vi "RT Main R2.vi"() -> ()   [LabVIEW 2018]
uses:
  Type Defs/Control Mode Type Def.ctl
  Type Defs/Sine Wave Inputs.ctl
  Type Defs/Measurement States.ctl
  <vilib>/Platform/TimedLoop/XDataNode/timing_clust.ctl
  <vilib>/Platform/TimedLoop/XDataNode/nitl_modes.ctl
  <vilib>/Platform/TimedLoop/XDataNode/wakeup.ctl
  Type Defs/PID Inputs.ctl
  <vilib>/FPGAPlugInAG/myRIO-1900/niLvFpga_Open_myRIO-1900.vi
  <vilib>/rvi/interface/common/dynamic/niFpgaDynamicAddResources.vi
  <vilib>/Utility/error.llb/Error Cluster From Error Code.vi
  <vilib>/rvi/errors/niLvFpgaAdjustHostInterfaceError.vi
  <vilib>/addons/control/pid/pid.llb/PID (DBL).vi
  <vilib>/FPGAPlugInAG/Dynamic/niLvFpga_Close_Dynamic.vi
  <vilib>/platform/TimedLoop/XDataNode/XDataNode.xnode
  <vilib>/rvi/interface/nirviOpenFPGA/nirviOpenFPGA.xnode
  FPGA Bitfiles/WattBalanceRev1_FPGATarget_FPGAMain2_Xz9O4wfmq2I.lvbitx
  FPGA/FPGA Main.vi
  <vilib>/rvi/interface/nirviReadWriteControl/nirviReadWriteControl.xnode
  <vilib>/rvi/interface/nirviCloseFPGA/nirviCloseFPGA.xnode
  <vilib>/rvi/interface/Simulation/niFpgaSimulationCallBeginRW.vi
  <vilib>/Platform/TimedLoop/XDataNode/XDNodeRunTimeDep.lvlib
  <vilib>/addons/control/pid/NI_PID_pid.lvlib
  NiFpgaLv.dll
panel:
  out "fake calculation time left":u32=605349941
  in  "N data points":i32
  in  "Set Point (um)":dbl format="%.2f"
  in  "Measure":bool
  out "Finished Late":bool
  in  "Amplifier On/Off":bool=TRUE
  out "Voice Coil Input Voltage":dbl[](array[numeric]) format="%#.2g"
  out "Displacement (µm)":dbl[](array[numeric])=[-0.0244140625] format="%#.2g"
  out "Voice Coil Back EMF":dbl[](array[numeric])=[0.49609375] format="%#.2g"
  in  "Sine Wave\nInputs":T1={"Amplitude (um)"=300.0, "Period (sec)"=0.05, "Offset (um)"=200.0}
  in  "Manual Voice \nCoil Voltage":dbl format="%.2f"
  in  "Abort":bool
  in  "Control Mode":T2=enum."Manual"
  out "Chart":dynamicdata(graph)=[{"t0"=timestamp(3604282469.873677 s since 1904-01-01), "dt"=1.0, "Y"=[0.0]}, {"t0"=timestamp(3604282469.873677 s since 1904-01-01), "dt"=1.0, "Y"=[-0.0244140625]}, {"t0"=timestamp(3604282469.873677 s since 1904-01-01), "dt"=1.0, "Y"=[0.49609375]}] caption="Waveform Chart - dark"
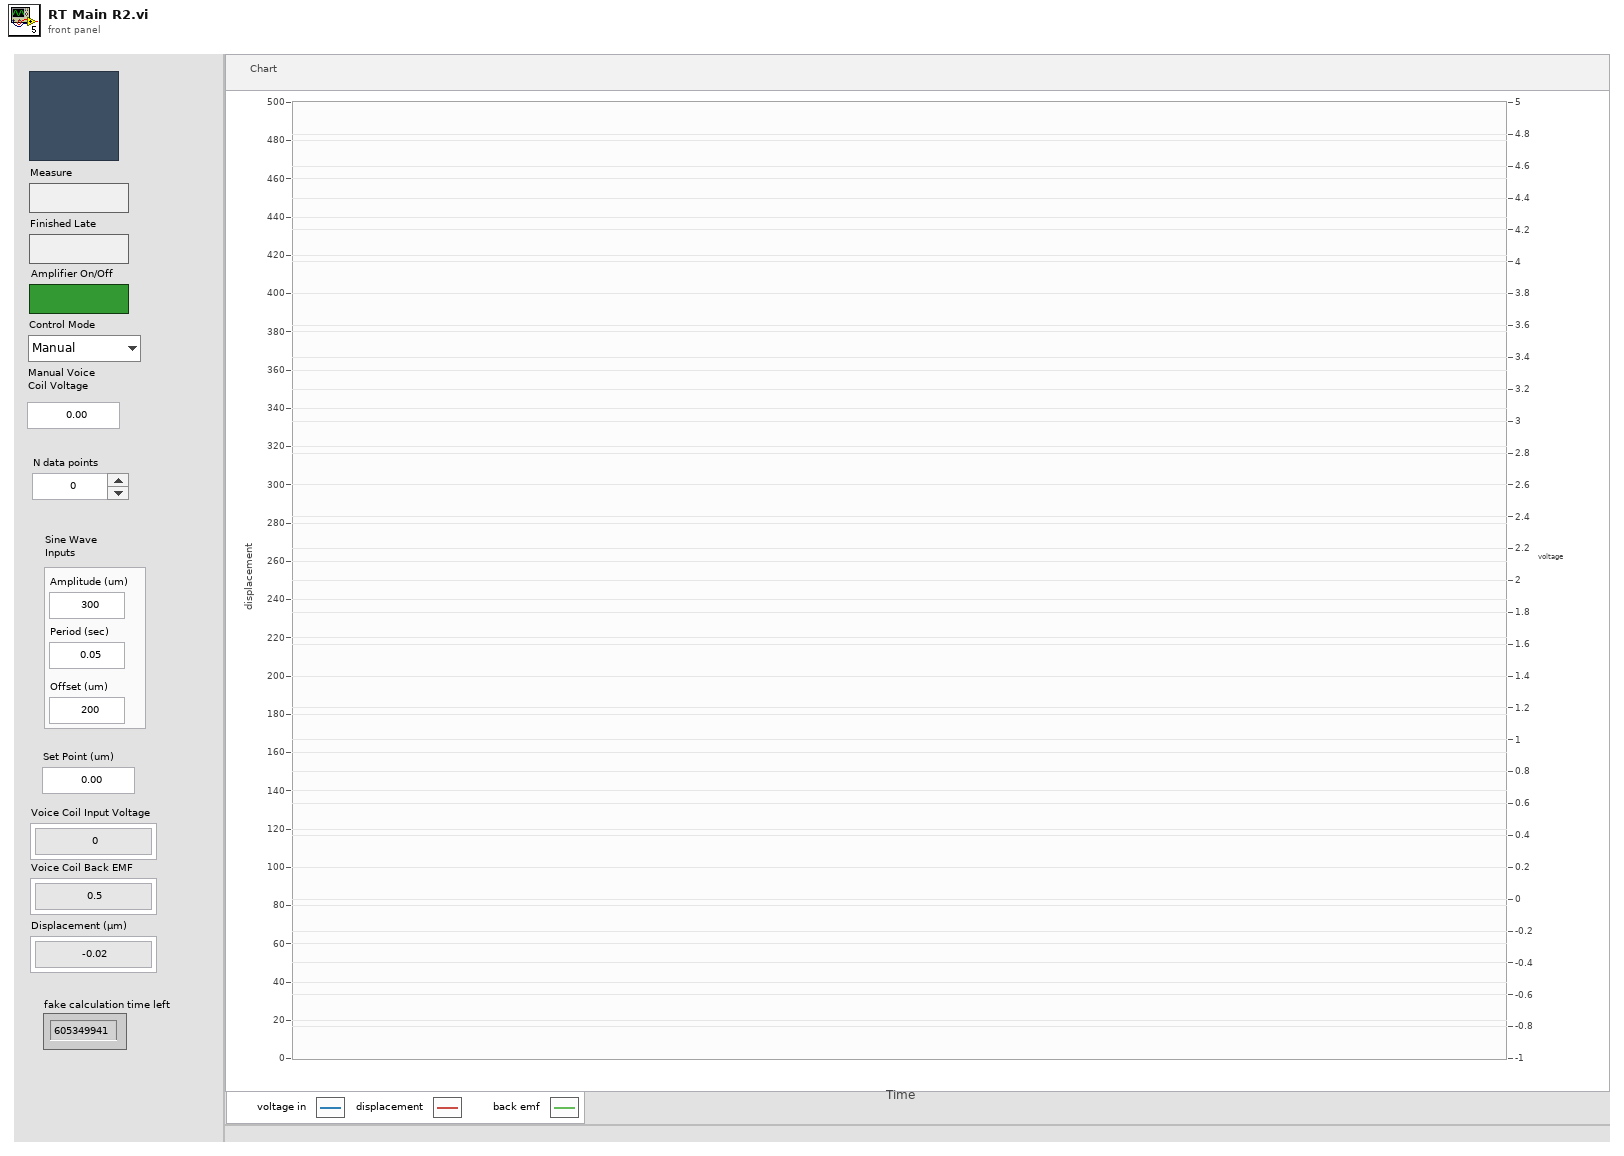
[diagram p1: front panel]
types:
  T1 = typedef "Sine Wave Inputs.ctl" = cluster{"Amplitude (um)":dbl, "Period (sec)":dbl, "Offset (um)":dbl}
  T2 = typedef "Control Mode Type Def.ctl" = enum16{"PID", "Manual"}
  T3 = typedef "Measurement States.ctl" = enum16{"Idle", "Initialize", "Collect Data", "Calculate", "Close"}
  T4 = typedef "XDNodeRunTimeDep.lvlib/timing_clust.ctl" = cluster{"Expected End [f-1]":u64, "Actual End [f-1]":u64, "Finished Late? [f-1]":bool, "Expected End [i-1]":u64, "Actual End [i-1]":u64, "Finished Late? [i-1]":bool, "Expected Start [i]":u64, "Actual Start [i]":u64, "Expected Start [f]":u64, "Actual Start [f]":u64, "Source Name":string, "Structure Name":string, "Period":i64, "Deadline":i64, "Offset":i64, "Start":i64, "Priority":i32, "Timeout":i32, "Mode":T5, "Wakeup Reason":T6, "Error":errorcluster, "Source Type":string, "Secondary Source Type":string, "Global End Time":u64, "Global Start Time":u64, "Frame Duration":u64, "Iteration Duration":u64, "Assigned CPU":i32, "I/O Scan Engine Mode":u32}
  T5 = typedef "XDNodeRunTimeDep.lvlib/nitl_modes.ctl" = enum32{"No Change", "Process missed periods, maintain original phase", "Discard missed periods, maintain original phase", "Process missed periods, ignore original phase", "Discard missed periods, ignore original phase"}
  T6 = typedef "XDNodeRunTimeDep.lvlib/wakeup.ctl" = enum32{"Normal", "Aborted", "Asynchronous wakeup", "Timing source error", "Timed loop error", "Timeout"}
  T7 = typedef "PID Inputs.ctl" = cluster{"PID":cluster{"Kp":dbl, "Ki":dbl, "Kd":dbl}, "Voltage Limits":cluster{"Max Voltage":dbl, "Min Voltage":dbl}, "Set Point (µm)":dbl}
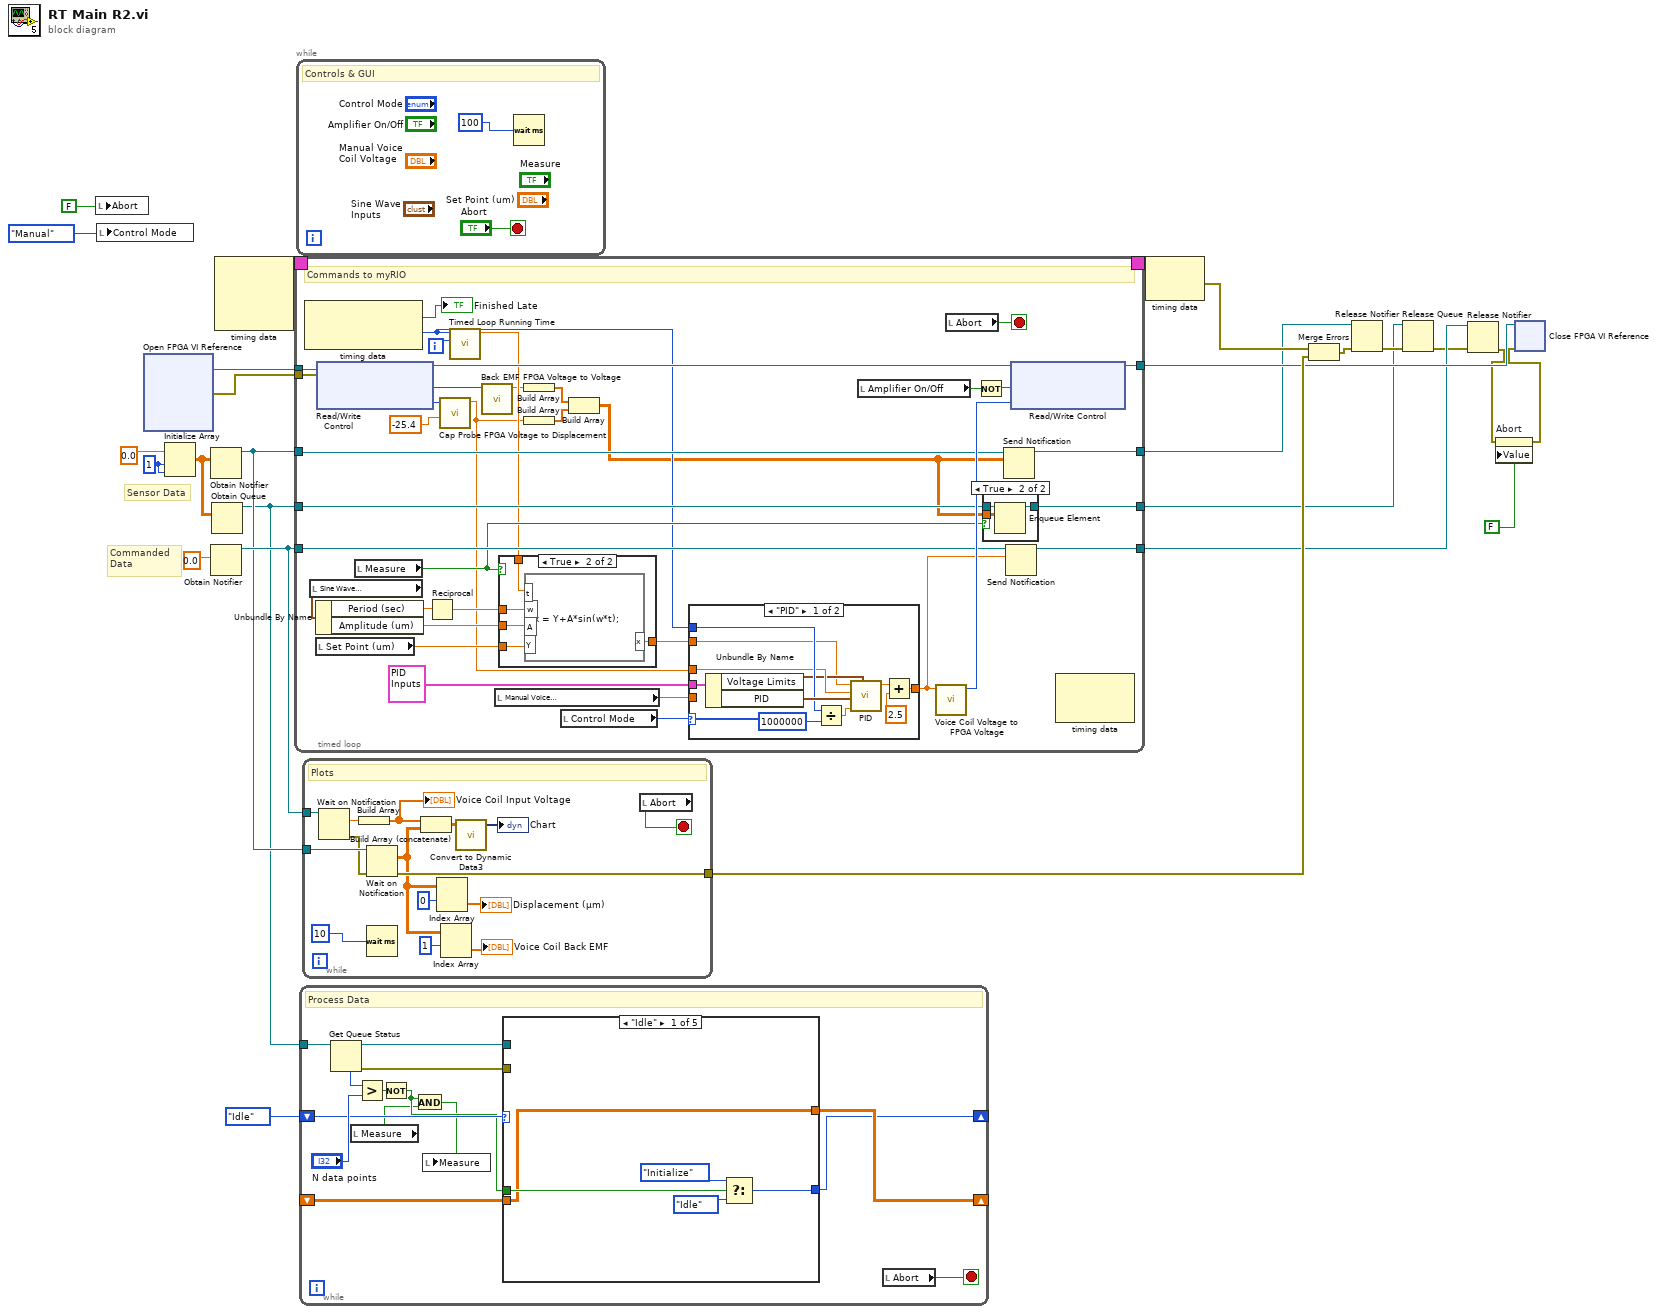
[diagram p0: block diagram]
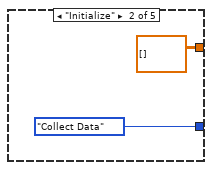
[diagram p2: hidden frame]
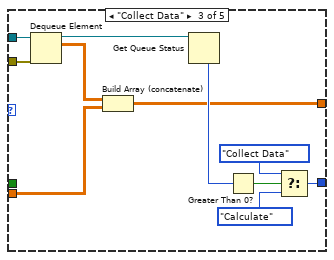
[diagram p3: hidden frame]
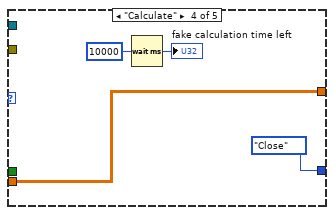
[diagram p4: hidden frame]
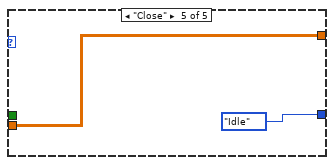
[diagram p5: hidden frame]
diagram:
  w22 = 1 ("dimension size")
  # "Commanded\nData"
  # "Sensor Data"
  n1 = local write "Abort"(FALSE) -> ()
  n2 = local write "Control Mode"(Control_Mode_Type_Def."Manual" ("Control Mode")) -> ()
  n3 = xnode "Open FPGA VI Reference"() -> ("FPGA VI Reference Out"=w24:refnum<k20>, "error out"=w5:errorcluster)  [unwired: 2 in]
  n4 = Initialize Array(0.0, w22, w22) -> (w14:dbl[][])
  n5 = Obtain Notifier(notification data type=w14) -> (notifier out=w10:refnum<notifier>)  [unwired: 3 in, 2 out]
  n6 = Obtain Notifier(notification data type=0.0) -> (notifier out=w17:refnum<notifier>)  [unwired: 3 in, 2 out]
  n7 = Obtain Queue(element data type=w14) -> (queue out=w9:refnum<queue>)  [unwired: 4 in, 2 out]
  n8 = node-c288() -> (w26:T4)  [unwired: 3 in]
  n9 = timed-loop {
    timing: w26 -> [_]
    timing-out: [_] -> w25
    tunnel: w24 -> [w52]
    tunnel: [w59] -> w18
    tunnel: w17 -> [w55]
    tunnel: [w53] -> w15
    tunnel: w10 -> [w51]
    tunnel: w9 -> [w50]
    tunnel: [w49] -> w7
    tunnel: [w48] -> w8
    tunnel: w5 -> [w46]
    i -> [w58]
    stop <- w60 stop-if-true
    # "Commands to myRIO"
    n10 = node-c288() -> (→"Finished Late":bool, w36:i64)  [unwired: 1 in]
    n11 = local read "Sine Wave\nInputs"() -> (w43:T1)
    n12 = Unbundle By Name(w43) -> ("Period (sec)"=w42:dbl, "Amplitude (um)"=w40:dbl)
    n13 = local read "Set Point (um)"() -> (w37:dbl)
    n14 = xnode "Read/Write Control"("FPGA VI Reference In"=w52, "error in"=w46) -> ("FPGA VI Reference Out"=w47:refnum<k20>, "Read Coil"=w33:i16, "Cap Probe Voltage"=w32:u16)  [unwired: 1 out]
    n15 = local read "Measure"() -> (w44:bool)
    n16 = Reciprocal(x=w42) -> (1/x=w41:dbl)
    n17 = call "Cap Probe FPGA Voltage to Displacement.vi"("Micrometers per Volt"=-25.4, "Cap Probe FPGA Voltage"=w32) -> ("Cap Probe Displacement"=w30:dbl)  [unwired: 9 in]
    n18 = call "Timed Loop Running Time.vi"("Counter"=w58, "Period (microsec)"=w36) -> ("Time (sec)"=w39:dbl)  [unwired: 9 in]
    n19 = call "Back EMF FPGA Voltage to Voltage.vi"("Back EMF In"=w33) -> ("Back EMF Out"=w31:dbl)  [unwired: 10 in]
    n20 = local read "Manual Voice \nCoil Voltage"() -> (w61:dbl)
    n21 = case shown="True" w44 {
      tunnel: [w64 w66] -> w45
      tunnel: w41 -> [_ w69]
      tunnel: w40 -> [_ w68]
      tunnel: w39 -> [_ w67]
      tunnel: w37 -> [w64 w65]
      frame False {
      }
      frame True {
        n22 = formula code="x = Y+A*sin(w*t);"("w"=w69, "t"=w67, "A"=w68, "Y"=w65) -> ("x"=w66:dbl)
      }
    }
    n23 = Build Array(w31) -> (w28:dbl[])
    n24 = Build Array(w30) -> (w29:dbl[])
    n25 = local read "Control Mode"() -> (w63:T2)
    n26 = Build Array(w28, w29) -> (w27:dbl[][])
    n27 = case shown="\"PID\"" w63 {
      tunnel: [w81 w89] -> w54
      tunnel: w61 -> [_ w89]
      tunnel: T7 {"PID"={"Kp"=-0.001, "Ki"=-0.001, "Kd"=0.0}, "Voltage Limits"={"Max Voltage"=1.0, "Min Voltage"=-1.0}, "Set Point (µm)"=200.0} ("PID Inputs") -> [w88 _]
      tunnel: w30 -> [w80 _]
      tunnel: w36 -> [w86 _]
      tunnel: w45 -> [w78 _]
      frame "PID" {
        n28 = Unbundle By Name(w88) -> ("Voltage Limits"=w79:cluster{"Max Voltage":dbl, "Min Voltage":dbl}, "PID"=w87:cluster{"Kp":dbl, "Ki":dbl, "Kd":dbl})
        n29 = Divide(x=w86, y=1000000) -> (x/y=w84:dbl)
        n30 = call-poly <vilib>:"PID.vi"("output range"=w79, "dt (s)"=w84, "PID gains"=w87, "process variable"=w80, "setpoint"=w78) -> ("output"=w82:dbl)  [unwired: 5 in, 1 out]
        n31 = Add(x=w82, y=2.5) -> (x+y=w81:dbl)
      }
      frame "Manual" {
      }
    }
    n32 = local read "Amplifier On/Off"() -> (w62:bool)
    n33 = call "Voice Coil Voltage to FPGA Voltage.vi"("Voltage In"=w54) -> ("Voltage Out"=w56:u16)  [unwired: 10 in]
    n34 = local read "Abort"() -> (w60:bool)
    n35 = Not(x=w62) -> (.not. x?=w57:bool)
    n36 = case shown="True" w44 {
      tunnel: [w70 w73] -> w49
      tunnel: w50 -> [w70 w72]
      tunnel: w27 -> [_ w71]
      frame False {
      }
      frame True {
        n37 = Enqueue Element(queue=w72, element=w71) -> (queue out=w73:refnum<queue>)  [unwired: 2 in, 2 out]
      }
    }
    n38 = Send Notification(notification=w27, notifier=w51) -> (notifier out=w48:refnum<notifier>)  [unwired: 1 in, 1 out]
    n39 = Send Notification(notification=w54, notifier=w55) -> (notifier out=w53:refnum<notifier>)  [unwired: 1 in, 1 out]
    n40 = xnode "Read/Write Control"("FPGA VI Reference In"=w47, "Amplifier On/Off"=w57, "Voice Coil Voltage"=w56) -> ("FPGA VI Reference Out"=w59:refnum<k20>)  [unwired: 1 in, 1 out]
    n41 = node-c288() -> ()  [unwired: 2 in, 1 out]
  }
  n42 = while {
    stop <- "Abort" stop-if-true
    # "Controls & GUI"
    n43 = Wait (ms)(milliseconds to wait=100) -> ()  [unwired: 1 out]
  }
  n44 = while {
    tunnel: w9 -> [w104]
    shift-right: [w97] -> _
    shift-left: _ -> [w98]
    shift-right: [w95] -> _
    shift-left: Measurement_States."Idle" -> [w96]
    stop <- w105 stop-if-true
    # "Process Data"
    n45 = Get Queue Status(queue=w104) -> (queue out=w103:refnum<queue>, error out=w102:errorcluster, # elements in queue=w101:i32)  [unwired: 2 in, 5 out]
    n46 = local read "Measure"() -> (w92:bool)
    n47 = Greater?(x=w101, y="N data points") -> (0:w99:bool)
    n48 = Not(x=w99) -> (.not. x?=w94:bool)
    n49 = And(x=w94, y=w92) -> (x .and. y?=w93:bool)
    n50 = local write "Measure"(w93) -> ()
    n51 = case shown="\"Idle\"" w96 {
      tunnel: [w109 Measurement_States."Collect Data" w121 Measurement_States."Close" Measurement_States."Idle"] -> w95
      tunnel: w103 -> [_ _ w120 _ _]
      tunnel: w102 -> [_ _ w119 _ _]
      tunnel: w94 -> [w108 _ _ _ _]
      tunnel: w98 -> [w106 _ w114 w126 w128]
      tunnel: [w106 dbl[][] [] w113 w126 w128] -> w97
      frame "Idle" {
        n52 = Select(t=Measurement_States."Initialize", s=w108, f=Measurement_States."Idle") -> (s? t:f=w109:T3)
      }
      frame "Initialize" {
      }
      frame "Collect Data" {
        n53 = Dequeue Element(queue=w120, error in (no error)=w119) -> (queue out=w118:refnum<queue>, element=w115:dbl[][])  [unwired: 1 in, 2 out]
        n54 = Build Array (concatenate)(w115, w114) -> (w113:dbl[][])
        n55 = Get Queue Status(queue=w118) -> (# elements in queue=w117:i32)  [unwired: 2 in, 7 out]
        n56 = Greater Than 0?(x=w117) -> (x > 0?=w116:bool)
        n57 = Select(t=Measurement_States."Collect Data", s=w116, f=Measurement_States."Calculate") -> (s? t:f=w121:T3)
      }
      frame "Calculate" {
        n58 = Wait (ms)(milliseconds to wait=u32 10000) -> (millisecond timer value=→"fake calculation time left":u32)
      }
      frame "Close" {
      }
    }
    n59 = local read "Abort"() -> (w105:bool)
  }
  n60 = while {
    tunnel: w10 -> [w143]
    tunnel: [w137] -> w20
    tunnel: w17 -> [w136]
    stop <- w144 stop-if-true
    # "Plots"
    n61 = Wait on Notification(notifier=w136) -> (notification=w134:dbl, error out=w135:errorcluster)  [unwired: 3 in, 2 out]
    n62 = Build Array(w134) -> (w133:dbl[])
    "Voice Coil Input Voltage" <- w133
    n63 = Wait on Notification(notifier=w143, error in (no error)=w135) -> (notification=w131:dbl[][], error out=w137:errorcluster)  [unwired: 2 in, 2 out]
    n64 = Wait (ms)(milliseconds to wait=10) -> ()  [unwired: 1 out]
    n65 = Build Array (concatenate)(w133, w131) -> (w132:dbl[][])
    n66 = Index Array(array=w131, index (row)=0) -> (element=→"Displacement (µm)":dbl[])  [unwired: 1 in]
    n67 = Index Array(array=w131, index (row)=1) -> (element=→"Voice Coil Back EMF":dbl[])  [unwired: 1 in]
    n68 = call "Convert to Dynamic Data3"("2D Array"=w132) -> ("Dynamic Data Type"=→"Chart":dynamicdata)  [unwired: 3 in]
    n69 = local read "Abort"() -> (w144:bool)
  }
  n70 = node-c288(w25) -> (w21:errorcluster)
  n71 = Merge Errors(w21, w20) -> (w19:errorcluster)
  n72 = Release Notifier(notifier=w8, error in (no error)=w19) -> (error out=w13:errorcluster)  [unwired: 1 in, 2 out]
  n73 = Release Queue(queue=w7, error in (no error)=w13) -> (error out=w12:errorcluster)  [unwired: 1 in, 2 out]
  n74 = Release Notifier(notifier=w15, error in (no error)=w12) -> (error out=w2:errorcluster)  [unwired: 1 in, 2 out]
  n75 = property on="Abort" class="Bool (strict)"(error in=w2, "Value"=FALSE) -> (error out=w1:errorcluster)  [unwired: 1 in, 1 out]
  n76 = xnode "Close FPGA VI Reference"("FPGA VI Reference In"=w18, "error in"=w1) -> ()  [unwired: 1 out]
